vi "Actor Core.vi"(8 "error in":errorcluster, 11 "Nested in":refnum<class "UserConsole.lvclass">) -> (0 "error out":errorcluster, 3 "Actor out":refnum<class "Actor.lvclass">)   [LabVIEW 2025, in "UserConsole.lvlib" / "UserConsole.lvclass"]
doc: "(<B>Filename</B>: Actor Framework.lvlib:Actor.lvclass:Actor Core.vi)\n\nReceives messages to the actor, reacts to them, and initiates any error handling that may shut the actor down.\n\nDescendant classes may override this VI to append parallel tasks for the actor to complete while it handles messages. Overrides use the Call Parent Method node."
uses:
  UserConsole.lvclass
  <vilib>/ActorFramework/Actor/Actor.lvclass
  <vilib>/ActorFramework/Actor/Actor.lvclass/Actor.ctl
  <vilib>/ActorFramework/Message Enqueuer/Message Enqueuer.lvclass/Message Enqueuer.ctl
  UserConsole.lvclass/UserConsole.ctl
  <vilib>/ActorFramework/Message Enqueuer/Init from Existing Queue.vi
  <vilib>/ActorFramework/Message Enqueuer/Enqueue.vi
  <vilib>/ActorFramework/Stop Msg/Stop Msg.lvclass
  <vilib>/ActorFramework/Message Priority Queue/Priority Enqueue.vi
  <vilib>/ActorFramework/Message Enqueuer/Message Enqueuer.lvclass
  C:/Program Files (x86)/National Instruments/LabVIEW 2025/vi.lib/ActorFramework/Actor/Actor.lvclass
  C:/Users/halstead_rideriver/Documents/Labview_Practice/ATM_Machine_Actor Framework/ATM_ACTOR_Without_States/UserConsole/UserConsole.lvclass
panel:
  out "Display2":string
  in  "USER CONSOLE :":T1
  in  "TRANSACTIONS:":T2
  in  "Card Reader":bool
  # "USER CONSOLE"
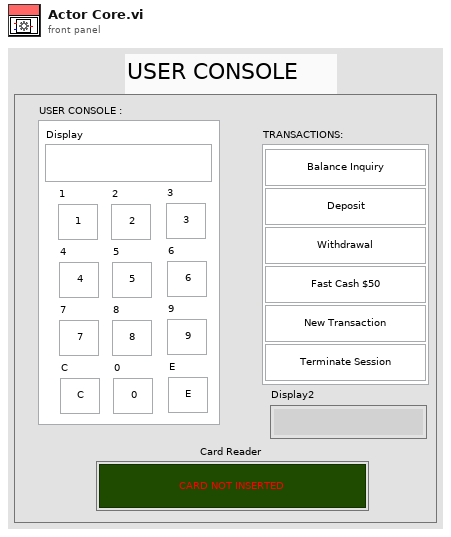
[diagram p1: front panel]
types:
  T1 = cluster{"1":bool, "2":bool, "3":bool, "4":bool, "5":bool, "6":bool, "7":bool, "8":bool, "9":bool, "C":bool, "0":bool, "E":bool, "Display":string}
  T2 = cluster{"Balance Inquiry":bool, "Deposit":bool, "Withdrawal":bool, "Fash Cash $50":bool, "New Transaction":bool, "Terminate Session":bool}
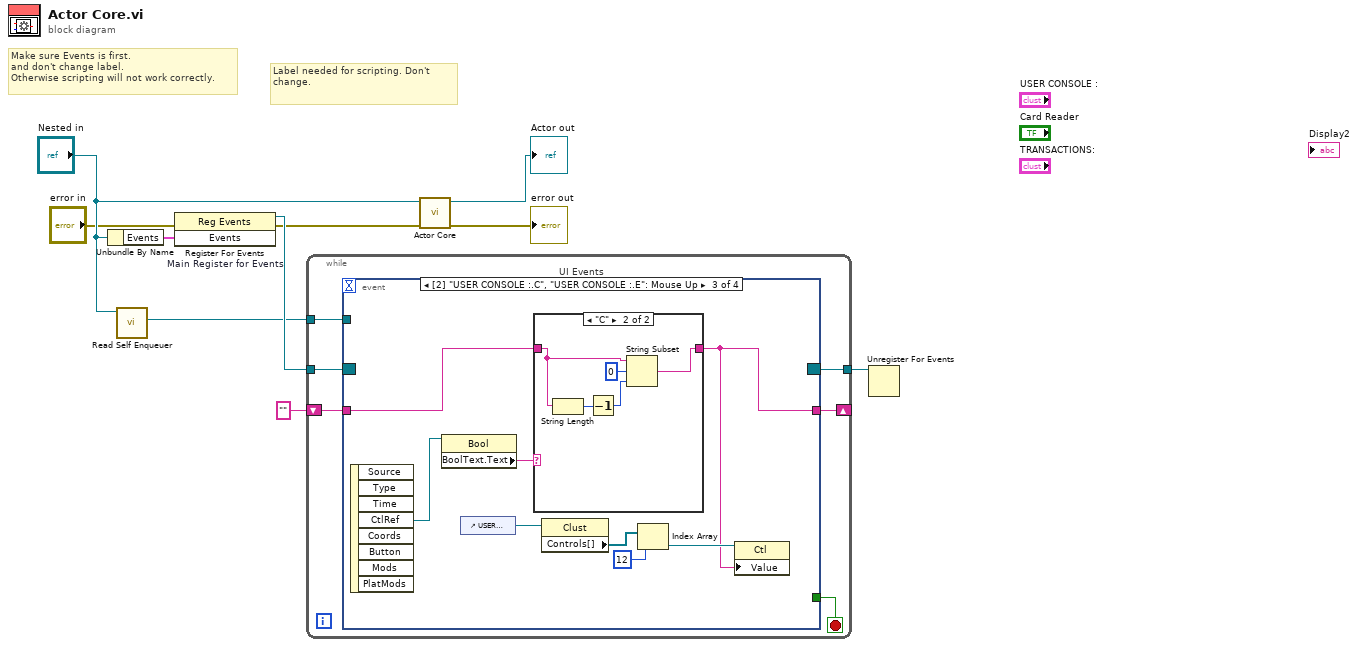
[diagram p0: block diagram]
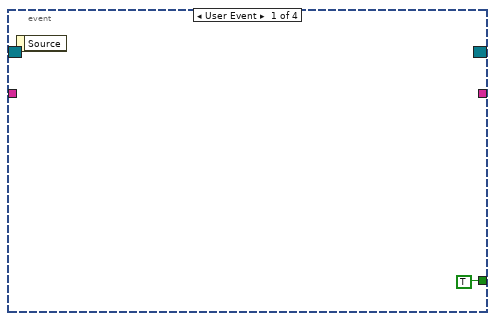
[diagram p2: hidden frame]
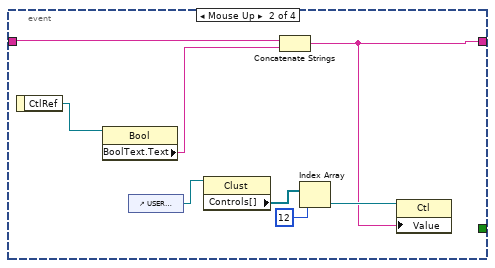
[diagram p3: hidden frame]
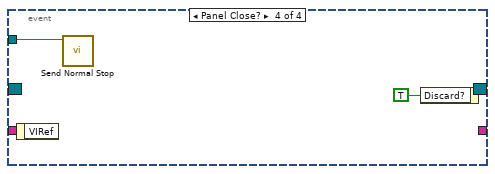
[diagram p5: hidden frame]
diagram:
  # "Label needed for scripting. Don't change."
  # "Make sure Events is first.\nand don't change label.\nOtherwise scripting will not work correctly."
  n1 = Unbundle By Name("Nested in") -> ("Events"=w7:cluster{"Stop":refnum<user-event>})
  n2 = call <vilib>:"Read Self Enqueuer.vi"("Actor"="Nested in") -> ("Self Enqueuer"=w4:refnum<class "Message Enqueuer.lvclass">)  [unwired: 10 in]
  n3 = register-events "Main Register for Events"(error in="error in", w7) -> (reference out=w8:refnum<event-registration>, error out=w2:errorcluster)  [unwired: 1 in]
  n4 = while {
    tunnel: w8 -> [w16]
    tunnel: [w14] -> w6
    tunnel: w4 -> [w13]
    shift-right: [w11] -> _
    shift-left: "" -> [w12]
    stop <- w15 stop-if-true
    n5 = event "UI Events" shown="[2] \"USER CONSOLE :.C\", \"USER CONSOLE :.E\": Mouse Up" {
      selector: w16 -> [_ _ _ _]
      dyn-events: [_ _ _ _] -> w14
      timeout: _ -> [_ _ _ _]
      tunnel: [TRUE _ _ _] -> w15
      tunnel: w13 -> [_ _ _ w40]
      tunnel: w12 -> [_ w20 w28 _]
      tunnel: [_ w19 w27 _] -> w11
      event User Event {
        n6 = event-data() -> ()  [unwired: 1 in, 1 out]
      }
      event "USER CONSOLE :.1", "USER CONSOLE :.2", "USER CONSOLE :.3", "USER CONSOLE :.4", "USER CONSOLE :.5", "USER CONSOLE :.6", "USER CONSOLE :.7", "USER CONSOLE :.8", "USER CONSOLE :.9", "USER CONSOLE :.0": Mouse Up {
        n7 = event-data() -> ("CtlRef"=w18:refnum<vi>)  [unwired: 1 in]
        n8 = property class="Bool"(reference=w18) -> ("BoolText.Text"=w22:string)  [unwired: 1 in, 2 out]
        n9 = control-ref of="USER CONSOLE :"() -> (w23:refnum<vi>)
        n10 = property class="Clust"(reference=w23) -> ("Controls[]"=w24:refnum<vi>[])  [unwired: 1 in, 2 out]
        n11 = Concatenate Strings(w20, w22) -> (w19:string)
        n12 = Index Array(array=w24, index=12) -> (element=w25:refnum<vi>)
        n13 = property class="Ctl"(reference=w25, "Value"=w19) -> ()  [unwired: 1 in, 2 out]
      }
      event "USER CONSOLE :.C", "USER CONSOLE :.E": Mouse Up {
        n14 = event-data() -> ("CtlRef"=w26:refnum<vi>)  [unwired: 1 in, 7 out]
        n15 = property class="Bool"(reference=w26) -> ("BoolText.Text"=w30:string)  [unwired: 1 in, 2 out]
        n16 = control-ref of="USER CONSOLE :"() -> (w33:refnum<vi>)
        n17 = case shown="\"C\"" w30 {
          tunnel: w28 -> [w34 w38]
          tunnel: [w34 w36] -> w27
          frame "E", Default {
          }
          frame "C" {
            n18 = String Length(string=w38) -> (length=w39:i32)
            n19 = Decrement(x=w39) -> (x-1=w37:i32)
            n20 = String Subset(string=w38, offset (0)=0, length (rest)=w37) -> (substring=w36:string)
          }
        }
        n21 = property class="Clust"(reference=w33) -> ("Controls[]"=w31:refnum<vi>[])  [unwired: 1 in, 2 out]
        n22 = Index Array(array=w31, index=12) -> (element=w32:refnum<vi>)
        n23 = property class="Ctl"(reference=w32, "Value"=w27) -> ()  [unwired: 1 in, 2 out]
      }
      event Panel Close? {
        n24 = event-data() -> ()  [unwired: 1 in, 1 out]
        n25 = call <vilib>:"Send Normal Stop.vi"("Message Enqueuer"=w40) -> ()  [unwired: 10 in, 1 out]
        n26 = event-data("Discard?"=TRUE) -> ()  [unwired: 1 in, 1 out]
      }
    }
  }
  n27 = call-parent "Actor Core.vi"("error in"=w2, "Actor in"="Nested in") -> ("error out"=→"error out":errorcluster, "Actor out"=→"Actor out":refnum<class "Actor.lvclass">)  [unwired: 8 in]
  n28 = Unregister For Events(event registration refnum=w6) -> ()  [unwired: 1 in, 1 out]
